vi "image.vi"() -> ()   [LabVIEW 2013]
uses:
  <vilib>/Analysis/Matrix/NI_Matrix.lvlib
  <vilib>/Utility/file.llb/Write To Spreadsheet File (DBL).vi
  <vilib>/Analysis/Matrix/Datatypes/RealMatrix.ctl
  <vilib>/Analysis/Matrix/Numeric/Conversions/Matrix To Array - RM.vi
  <vilib>/Utility/file.llb/Read From Spreadsheet File (DBL).vi
panel:
  in  "Normalize?":bool
  in  "Save The Cross Section":bool
  in  "ON":path=path "/Macintosh HD/Users/Ruchira/Desktop/scan1/ON1/Y-32_fit.txt"
  in  "OFF":path=path "/Macintosh HD/Users/Ruchira/Desktop/scan1/ON1/y_31_fit.txt"
  out "Intensity Graph":dbl[][](graph)=[[0.0999961901429774], [0.10000123166150422], [0.10000135033082976], [0.09999704994321655], [0.09999759071413349], [0.10000084663946385], [0.1000012117498761], [0.10000097689275309], [0.10000164876308568], [0.09999648287738241], [0.10000110689586153], [0.09999818237676397], [0.10000126793860856], [0.09999754550814881], [0.0999980392905063], [0.10000044482376341], [0.09999913803857505], [0.10000050220417034], [0.09999715423524554], [0.09999799513810394], [0.10000181351533373], [0.09999709728037659], [0.09999777905934876], [0.09999707127163737], [0.10000127901557891], [0.09999796410448629], [0.09999718267251918], [0.0999985636671887], [0.09999841240954438], [0.09999808500763945], [0.10000238691137875], [0.10000161846358738], [0.09999822930044115], [0.10000075848082599], [0.10000068933923355], [0.1000024236518158], [0.10000290568154932], [0.10000085686473831], [0.10000230225985311], [0.10000149836735855], [0.09999986636917042], [0.10000359405031024], [0.10000312564210484], [0.10000313147057305], [0.10000118234594123], [0.09999987554916473], [0.10000181684992422], [0.10000185606097113], [0.1000025842332808], [0.10000227930825865], [0.10000347944496162], [0.10000100625483241], [0.10000142101694179], [0.10000314994033971], [0.10000154469593482], [0.10000192220644337], [0.10000466479003443], [0.10000234032096383], [0.10000240345292899], [0.10000149911732752], [0.09999740374791438], [0.10000136412307498], [0.10000352573058052], [0.1000004648002058], [0.10000005079292161], [0.09999955770073203], [0.10000069450692534], [0.10000304014390352], [0.10000122773941927], [0.10000168512743678], [0.10000194792402127], [0.10000192695259297], [0.09999968237859753], [0.09999958623911322], [0.10000118777877205], [0.1000020603567743], [0.10000218588046038], [0.09999977985541698], [0.09999861297897399], [0.09999954403466309], [0.09999933084000477], [0.09999924980119886], [0.10000027299563718], [0.10000009189068723], [0.10000110682583423], [0.10000077949470162], [0.10000090534418594], [0.10000018726331182], [0.10000096980436052], [0.09999980494871381], [0.10000015878968854], [0.09999959204869212], [0.09999941000101689], [0.09999977355307214], [0.09999859679949125], [0.09999840143639106], [0.10000016454514019], [0.10000045652323415], [0.10000047732317208], [0.10000020087238798], [0.09999882340527957], [0.10000007126845203], [0.10000029214685592], [0.09999925931062281], [0.09999926329087266], [0.09999907646140645], [0.09999858993485494], [0.09999968917439243], [0.09999913973681834], [0.09999875844725434], [0.09999896445513062], [0.09999900543682053], [0.09999993071718452], [0.0999999102386502], [0.0999995214120633], [0.09999971735154342], [0.09999950486441825], [0.09999880162641392], [0.09999922584335166], [0.09999956823609847], [0.09999999668927682], [0.09999992113306001], [0.09999971240104609], [0.09999961415606441], [0.0999990191996489], [0.09999954251806992], [0.09999925150144613], [0.0999998365982448], [0.09999958671879616], [0.09999910599373554], [0.09999996361215446], [0.09999957627411026], [0.09999995030056676], [0.09999968902034741], [0.09999996957666005], [0.09999974435093766], [0.09999976482429569], [0.10000003037414487], [0.09999998475569946], [0.09999954938348765], [0.09999979074987307], [0.09999965366084819], [0.10000001991255952], [0.1000001850647135], [0.09999985563509438], [0.09999995855033227], [0.09999976121025504], [0.09999937741961164], [0.09999998666441115], [0.10000015954726275], [0.1000004123670828], [0.1000001063637803], [0.09999992798411764], [0.10000007921436647], [0.09999993517716374], [0.09999984988689666], [0.10000009355836353], [0.09999967891713826], [0.09999987103828216], [0.1000000712813875], [0.09999998747709593], [0.09999993295305948], [0.09999986632106737], [0.10000013745021331], [0.09999981188499174], [0.09999989255622112], [0.0999999919648023], [0.09999971354271445], [0.10000042793585165], [0.09999969311683246], [0.10000006809921125], [0.10000018404218568], [0.10000018015349744], [0.10000005384694884], [0.09999989767787482], [0.09999983532018687], [0.10000003722495465], [0.09999962269635267], [0.09999976172061785], [0.09999984532447814], [0.09999998784616544], [0.0999999039419567], [0.10000008441502968], [0.09999972051132222], [0.10000008779089652], [0.1000002890351282], [0.10000008731841208], [0.09999994222108334], [0.09999983237672086], [0.10000013421033312], [0.10000005141733095], [0.10000006535189712], [0.09999992565779832], [0.09999958959090645], [0.09999970593383432], [0.09999988681797735], [0.09999984714438878], [0.09999991710543132], [0.099999686490646], [0.0999998794498034], [0.09999985778736376]]
  in  "parameter Constrains":T1={"amp min"=-1.0, "amp max"=1.0, "center min"=600.0, "center max"=700.0, "FWHM min"=10.0, "FWHM max"=100.0, "offset min"=0.0, "offset max"=0.0}
  in  "File Format":u16(ring) items=["JPG", "PNG", "BMP"]
  in  "SigFig (micron)":dbl=1.0
  in  "Background Substract":bool=TRUE
  in  "Zoom Factor":sgl=1.0
  out "Picture":picture
  in  "path to bmp file":path=path "/Macintosh HD/Users/Ruchira/Desktop/ps.jpg"
  in  "Fitting Function":enum16{"Lorantzian", "fano", "gaussian"}(ring)=enum."gaussian"
  in  "Filter ?":bool=TRUE
  in  "?":u32(colorbox)=16715776
  in  "?":bool
  in  "?":u16(ring)=2 items=["", "Pick Spectrum ", "Fit Spectra", "Cross Section"]
  in  "?":bool
  in  "Fitting Directory":path=path "/Macintosh HD/Users/Ruchira/Desktop/scan1/ON1/Y_32_0/dia_1_X_39_4_Y_32_0_ON"
  in  "Initial \nparameters":dbl[](array[numeric])=[0.0, 0.1, 50.0, 183.0]
  out "Waveform Graph":cluster{"Array":dbl[]}[](graph)=[{"Array"=[0.999912, 1.0000062, 0.9999195, 1.0007249, 0.9996202, 0.9991244, 1.0002736, 0.9998005, 1.0002531, 1.0001882, 0.9997705, 0.9996142, 0.9994632, 0.9997326, 0.99964, 0.9993857, 1.0000215, 1.0006765, 0.9997504, 1.0006266, 0.9997772, 0.9992525, 1.0001104, 0.9999963, 0.9997144, 0.9990248, 0.99969, 0.9989677, 1.0008024, 0.9994781, 0.9996141, 0.9997979, 0.9997724, 0.9996542, 1.0000813, 0.9995505, 0.9997522, 0.9992789, 0.9997476, 1.0005772, 0.9997887, 0.9996226, 1.0004367, 1.0009052, 1.0000415, 0.9992441, 0.9992899, 0.9988662, 1.0001159, 0.9993691, 1.0000963, 0.998833, 0.9988622, 1.0002627, 0.9992917, 0.9994175, 0.9991441, 0.9992283, 0.9990043, 0.9988636, 1.0000361, 0.9996554, 0.9992461, 0.9990231, 0.999462, 0.9993146, 0.9997979, 1.0003636, 0.9998718, 0.999412, 0.9993142, 0.9986716, 0.9996698, 0.9993684, 0.9988869, 0.9991172, 1.0003158, 0.9997581, 1.0000962, 0.9996494, 0.9995781, 0.9989753, 0.9997771, 0.9995659, 0.9990109, 0.9994639, 0.9990328, 1.0002382, 0.9992761, 0.9996792, 0.9989703, 0.9994579, 0.9998822, 0.9984634, 0.9992488, 0.9996927, 0.9996856, 0.9999188, 0.9991421, 0.9996352, 0.9995514, 0.9994296, 0.9998158, 1.0003442, 0.9993032, 0.9998166, 0.9991794, 0.9992785, 0.9989296, 0.9992176, 0.9996715, 1.0002317, 0.9997447, 1.000023, 0.9999388, 1.0000318, 0.9993103, 0.9983221, 0.9997067, 0.9992942, 0.9994903, 1.000274, 0.9993993, 0.9996543, 0.9994589, 0.9987717, 0.9995216, 0.9996218, 0.9997857, 1.0003538, 1.0003287, 0.9998377, 1.0000575, 0.9994548, 0.999651, 1.000589, 0.9999774, 0.9998517, 0.9997108, 0.9997329, 0.9987114, 1.000017, 0.9998208, 0.9995178, 0.9995105, 0.9992935, 1.000017, 0.999771, 0.9997507, 0.9998368, 0.9989039, 0.9994854, 0.9991881, 0.9997416, 0.9995755, 0.9996139, 1.0004916, 0.9996789, 0.9997569, 1.0006737, 0.9995899, 0.9995284, 1.0003346, 0.9997696, 0.9997103, 0.9992941, 0.9995254, 0.9998266, 0.9995101, 0.999556, 0.9996889, 0.999612, 1.0004629, 0.9998417, 0.9998443, 0.9995054, 1.0001907, 0.999727, 1.0002715, 0.9998889, 0.9997173, 0.9996202, 0.9993741, 0.9997404, 0.9998444, 0.9995518, 0.9998645, 1.0002948, 0.9995542, 0.9993841, 0.9996716, 1.0003395, 0.9995428, 0.9992663, 0.9998679, 0.9990207, 0.9997029, 0.9999758, 1.0002127, 0.9991095, 0.9997171, 0.9994459, 0.9995794, 0.9996757, 0.9995238, 0.9992508, 0.9995349, 0.9996876, 0.9998513, 1.0002972, 1.0005107, 0.9995459, 0.9997344, 0.9993501, 0.998904, 0.9994265, 0.9996681, 0.9997693, 0.9998932, 1.0004375, 1.0003389, 0.9999753, 0.9999445, 1.0002389, 0.9992193, 1.0007039, 0.999621, 1.0005075, 0.9990674, 0.9989446, 0.9998963, 0.9995903, 0.999903, 0.9996576, 0.9997039, 0.9999802, 1.0004561, 0.9996246, 0.9994775, 1.0002422, 0.9993529, 1.0001368, 0.9998639, 1.0000355, 0.9992625, 0.9995799, 0.9999136, 0.9999445, 0.9994137, 1.0002099, 1.0002885, 0.9998356, 1.0008825, 1.0000316, 0.9999662, 0.9992243, 0.9998829, 1.0007041, 1.0002848, 0.9993363, 1.0001841, 1.0000274, 1.0003478, 1.0003174, 0.9999082, 1.0002834, 1.0002627, 0.9997852, 0.9991637, 1.0003098, 1.0002492, 1.0005535, 0.999675, 0.999759, 0.9995484, 1.0001614, 1.0000287, 1.0001989, 1.0004951, 1.0004172, 0.9999552, 0.9996557, 1.0003109, 0.9995099, 0.9997021, 0.9992045, 1.0007278, 0.9994112, 0.9999635, 0.9993279, 0.9996014, 1.0003337, 1.0000202, 0.9997986, 0.9991892, 0.9998672, 1.0000011, 0.9995615, 0.9991948, 0.9995186, 0.9998185, 0.9995575, 1.0000313, 0.9999638, 0.9999951, 1.0012059, 0.9997584, 1.0005391, 1.0011878, 1.000318, 0.9996395, 0.9996092, 0.9994599, 0.9997242, 1.0000628, 0.9993907, 0.9998052, 0.9995693, 1.0002239, 0.9993822, 0.9989864, 1.0008243000000001, 1.0008603, 1.000017, 0.99964, 0.9998918, 1.0009811, 0.9995773, 0.9999757, 0.9994455, 0.9999629, 0.9989937, 0.9993532, 0.9988021, 0.999775, 0.9994477, 1.0005354, 1.0004217, 0.9990068, 0.9990595, 0.999235, 0.9997253, 0.9999283, 1.0003691, 0.9987342, 0.9987156, 0.99932, 1.0006941, 0.9990174, 0.9995789, 1.0000781, 0.999864, 0.9987173, 0.9995567, 0.9998158, 0.9990578, 0.9997313, 0.9996173, 0.9997118, 1.0001294, 0.9995772, 0.9997848, 0.9992174, 1.0002083, 0.9998677, 0.999437, 0.9986994, 0.9989801, 0.9988885, 0.9988535, 0.9991101, 0.9993622, 1.0000297, 0.9998208, 0.9996366, 0.9999674, 0.9999051, 0.9994292, 0.9993126, 0.999776, 0.9990464, 0.9995287, 1.0005, 0.9994522, 0.9989594, 1.0000136, 0.998607, 0.9995734, 0.9998784, 0.9987946, 0.9995151, 0.9989061, 0.9996754, 0.9996827, 0.9990179, 0.9994808, 1.0005484, 0.9993381, 0.9996653, 0.9997457, 0.9998257, 0.9999206, 0.9996306, 0.9996981, 0.9994915, 1.000414, 0.9991374, 0.9999802, 0.9990244, 0.9995426, 0.9994226, 1.0005428, 0.9997184, 0.9996405, 0.9998817, 0.9990332, 0.999546, 0.9994692, 0.9995606, 0.999712, 1.0004374, 0.9985378, 1.0000077, 1.0013742, 0.9989422, 0.9999068, 0.999257, 0.9993879, 0.9996964, 1.0003505, 0.9998826, 0.9994893, 0.9999303, 1.000442, 1.0001266, 1.0005605, 0.9992218, 0.9994654, 0.9990975, 0.9999623, 0.9990798, 0.9998905, 0.9991768, 0.999592, 0.9999166, 0.9999282, 1.0001616, 1.0005988, 1.000266, 0.9993236, 1.0001337, 0.9993938, 0.9994889, 0.9982496, 1.0000666, 0.9995728, 0.9988732, 1.0000484, 0.9996128, 0.9998416, 0.9999103, 0.9994758, 0.9999986, 0.9992403, 0.9991495, 1.0000631, 0.9990761, 1.0002229, 1.0000052, 1.000004, 0.9996256, 1.0000775, 0.999592, 0.9997201, 0.9989163, 0.9989697, 1.0002479, 0.9999675, 0.999776, 0.9997987, 0.9994048, 0.9998939, 0.9997733, 0.9986924, 0.999714, 0.9994414, 1.0002745, 1.0000148, 0.9997425, 0.9995858, 1.0002273, 0.9996642, 1.0005309, 0.9997909, 0.9998647, 1.0004744, 0.9994365, 1.0003841, 1.0001789, 1.0003809, 0.9991066, 1.0002345, 1.0005149, 0.9986604, 1.0000528, 1.0003553, 0.9996183, 0.999854, 1.0004234, 0.9991074, 0.9999751, 0.9996607, 1.0001485, 1.00034, 0.9991534, 0.9996239, 0.9999622, 0.9999014, 0.9998442, 0.9994333, 0.9996824, 1.0012007, 0.9990924, 0.9996013, 0.9998479, 0.9997425, 0.9990558, 1.000082, 1.000111, 1.0005331, 1.0000641, 0.9994033, 1.0004079, 1.0001025, 1.0000838, 0.9990626, 1.0006284, 1.0000943, 1.000137, 0.9993611, 0.9996293, 1.0003729, 0.9998056, 1.0000649, 1.0002914, 0.9996269, 0.9997866, 0.9999594, 0.9997383, 0.9991266, 1.0001618, 0.9994388, 1.0002258, 0.9994914, 1.0000562, 0.9995762, 0.9998524, 0.9996511, 1.0010098, 0.9996345, 0.9992435, 0.9996726, 1.0001917, 1.0004534, 0.9996527, 0.9996541, 0.9994873, 0.998815, 0.9997382, 0.9989723, 0.9993279, 0.9988684, 1.0005942, 0.9979386, 0.9996604, 0.998509, 1.0000703, 0.999597, 0.9994641, 0.9995958, 0.999995, 0.9996274, 0.9998089, 0.9989087, 0.9996136, 1.0007132, 0.9995889, 0.99931, 0.9995004, 0.9986379, 0.99934, 0.9992054, 0.9991074, 1.0002335, 1.0002441, 0.999719, 0.9996165, 0.9997128, 0.998794, 0.9988396, 0.9998567, 0.9993354, 0.9993648, 0.9989801, 0.9996489, 0.9993824, 0.9998368, 0.9980654, 1.0000289, 0.9985257, 1.0002826, 0.999874, 0.9997462, 0.9995808, 0.9995395, 0.9988734, 0.9980803, 0.9995798, 1.00039, 0.9992561, 0.9996533, 0.9999288, 0.9985423, 0.9993574, 1.0003907, 0.9988179, 0.9996707, 0.9997962, 0.9988759, 1.0002284, 0.9996408, 0.9988728, 0.999683, 0.9994447, 1.0004125, 1.0008299, 0.9987556, 0.9992713, 0.9994446, 0.9983223, 0.9995367, 0.9980671, 0.9992592, 0.9998817, 0.9989496, 0.9996664, 1.000473, 0.9987348, 1.0003217, 0.9988259, 0.9988114, 1.0002154, 0.9995201, 0.9992665, 0.9992888, 0.9988897, 0.9986637, 0.9997617, 0.9991824, 0.998652, 0.999192, 0.9997019, 0.9985744, 0.9999023, 0.99976, 0.9989789, 0.9992547, 0.9985736, 1.0000799, 0.9994289, 1.000198, 1.0004209, 0.9995535, 0.9995055, 0.9999917, 0.9978965, 1.000103, 1.0002614, 0.9987275, 0.9997208, 0.9995843, 1.0004293, 0.9999196, 0.9997547, 0.9997684, 1.0000823, 0.9990606, 1.0000749, 1.0006261, 0.9992032, 1.0003915, 0.9986865, 0.9993972, 1.0006179, 0.999223, 0.9995273, 0.9999418, 0.9997804, 0.9990067, 0.9994214, 0.9988363, 0.9997792, 0.9992232, 0.9994337, 0.9996303, 0.9990614, 0.9987737, 0.9991485, 0.9999368, 0.9988097, 1.000023, 0.999718, 0.9993419, 0.9995108, 0.9988932, 0.9996122, 0.9996549, 0.9993274, 1.0007295, 0.9987502, 0.9991907, 1.000245, 0.9996555, 1.0001368, 0.9997992, 0.9998987, 0.9993079, 0.9997203, 1.0001504, 0.9991114, 0.9996201, 0.9997694, 0.998722, 0.9989102, 0.9998005, 0.9989434, 0.9990453, 1.0000478, 0.9993367, 0.9997115, 0.9999445, 0.998842, 0.9981667, 0.9997795, 0.9979156, 0.9987582, 0.9999457, 0.9985634, 0.9987168, 0.9989546, 0.9996025, 0.9987306, 0.9993737, 0.9990279, 0.9986008, 1.0004001, 0.9993854, 0.9993435, 0.9991244, 0.9991655, 0.9991997, 0.9996201, 0.999556, 0.9993827, 0.9996332, 0.9998294, 0.9992972, 0.9993395, 0.9992943, 0.9997331, 0.9996559, 0.9993133, 0.9997332, 1.0001546, 0.9998963, 0.9988493, 0.9982228, 0.9990334, 0.9996922, 0.999585, 0.99872, 0.9992144, 0.9997141, 0.998995, 1.0001988, 0.9992188, 0.9993191, 1.000408, 0.9996398, 0.9984199, 1.0003845, 0.9990073, 0.9987424, 0.9991647, 0.9990882, 1.0006108, 0.9996878, 0.9994017, 0.9997925, 0.9993464, 0.9995282, 1.0002015, 0.9995041, 0.9989298, 0.9996913, 0.998544, 0.9995248, 1.000274, 0.9993534, 0.9992568, 0.9998172, 0.9985249, 0.9998827, 0.9999777, 0.9996465, 0.9993267, 0.9985538, 0.9999634, 0.999692, 0.9998105, 0.9990786, 0.998777, 0.998742, 0.9994866, 0.9991291, 0.9991076, 0.9994755, 0.9993844, 0.9996325, 0.9997167, 0.9983325, 1.0000013, 1.0003206, 0.9993017, 1.0000534, 0.998928, 0.9992802, 1.0004163, 0.9985779, 0.9987091, 1.000012, 0.9995588, 0.9989666, 0.9986488, 0.9992081, 0.9996518, 1.0000042, 0.9990546, 0.9992699, 0.998815, 0.9993366, 0.9996229, 0.9992526, 0.9996555, 0.999927, 0.9989395, 1.0002995, 0.9994138, 0.9993524, 0.9989039, 0.9998021, 0.999467, 1.0003852, 0.9994779, 0.9991215, 1.0007633, 0.9992624, 0.999852, 0.999191, 0.9999406, 0.999067, 0.9998017, 0.9986019, 1.0000399, 0.9990516, 1.0003929, 0.9990066, 0.9995693, 0.9990149, 0.998768, 0.9999348, 0.9995828, 0.9993824, 0.9994241, 0.9989466, 0.9997066, 0.9991827, 1.0010118, 0.9997681, 0.9998445, 0.9988864, 0.9984717, 0.9995148, 0.9990124, 0.9994546, 0.9992063, 0.9994997, 0.9993552, 0.9985694, 0.9990449, 0.9988327, 0.9995954, 0.9989215, 0.9998563, 0.9991389, 0.9996583, 0.9996954, 0.9990346, 0.9989564, 0.9989618, 0.9990742, 0.9990664, 0.9993067, 0.999248, 0.9994816, 0.9991723, 0.9989503, 0.99956, 0.9992029, 0.9983765, 0.9996398, 0.9984304, 0.9994204, 1.0000248, 0.9995871, 0.9990603, 0.9995035, 0.9984536, 1.0001651, 1.0006427, 0.9989779, 0.9993951, 0.9994604, 0.9985639, 1.0000989, 0.998099, 0.9991217, 0.9990972, 0.999027, 0.9985814, 0.9985801, 0.9989235, 0.9996577, 0.9997086, 0.998898, 0.9996104, 0.9989361, 0.998648, 1.0002115, 0.9990118, 0.9988677, 0.9994482, 0.999177, 0.9990072, 0.9995065, 0.9993331, 0.9990698, 0.9986496, 0.9995377, 1.0006704, 0.9992097, 0.9987989, 0.9985685, 0.99976, 0.9987426, 0.9995563, 0.9991248, 0.9992443, 0.9989276, 0.9983766, 0.9994139, 0.9997891, 0.999956, 0.9992304, 0.9987388, 0.9984953, 0.999307, 0.9990246, 0.9988373, 0.9989017, 0.9991426, 0.9991718, 0.9992229, 0.9985943, 0.9989612, 0.9988095, 0.9995043, 0.9991213, 0.9993649, 0.9995521, 1.000257, 0.9991396, 0.9996828, 0.9988623, 0.9991661, 0.9982617, 0.9993377, 0.9976886, 1.0005162, 0.9987226, 0.9993491, 0.9984059, 0.998636, 0.999556, 0.9992717, 0.9984921, 0.999401, 0.9984477, 0.9991464, 1.0000037, 0.9990402, 0.9993154, 0.9992363, 0.9988391, 0.9996333, 0.9989477, 0.9992048, 1.0000735, 0.9992126, 0.9990736, 1.0003862, 0.9995333, 0.9994013, 0.9993385, 0.999072, 0.9992918, 0.9987017, 0.9996325, 0.9990081, 0.9996133, 0.9989096, 0.9989104, 0.9980355, 0.9995976, 0.9986304, 0.9988823, 0.9993512, 0.9986036, 0.9984648, 0.999202, 0.9995629, 0.9992173, 0.9987362, 0.9980147, 0.9998687, 0.9992276, 0.9989575, 0.998889, 0.9992327, 0.9991231, 0.9992699, 0.9997416, 0.9996087, 0.9996938, 0.9989509, 0.9993734, 0.9988294, 0.9991869, 0.9991652, 0.9986817, 0.999805, 0.9988091, 0.9987919, 0.9989816, 0.9995875, 0.9990158, 0.9986354, 0.9997111, 0.9997297, 0.9987274, 0.999885, 0.9991252, 0.9996094, 0.999989, 0.9991881, 0.9997831, 0.9996842, 0.9993126, 0.9997881, 0.9988679, 0.9990894, 0.9998617, 0.9991554, 0.9990344, 0.9992666, 0.9993193, 0.9999206, 0.9986974, 0.9992499, 1.0003586, 0.9988287, 0.9992303, 0.9998635, 0.9986143, 0.9980053, 1.0005758, 0.9976869, 0.9992939, 0.9987265, 0.9985804, 0.9985005, 0.9994571, 0.9989679, 0.9991719, 0.9984729, 0.9984019, 0.9995559, 0.9994761, 0.9997828, 0.9992282, 0.9989886, 0.9981934, 0.9990812, 0.998116, 0.9995994, 0.9989792, 0.9983792, 0.999598, 0.9988397, 0.9984028, 0.999649, 0.9988168, 0.9995654, 1.000411, 0.9986991, 0.9996752, 0.9986717, 0.9991131, 0.9988728, 0.9989572, 0.9981359, 0.9992972, 0.9988086, 0.9991376, 0.9990386, 0.9991565, 0.9990703, 0.9993521, 0.9986112, 1.0000715, 0.9986865, 0.9980398, 0.9988252, 0.9988827, 0.9982868, 0.999154, 0.9989643, 0.9991873, 0.998705, 0.9998231, 0.9993724, 0.9990766, 0.9987374, 0.9991775, 0.998257, 0.9984206, 1.0001665, 0.9987628, 0.9992235, 0.9991029, 0.9983892, 0.9999527, 0.9993111, 0.9989074, 0.999224, 0.9994221, 0.9993205, 0.9987931, 0.998174, 0.9995541, 0.9994415, 0.9990281, 0.9983542, 0.9989866, 0.999845, 0.9979003, 0.9987047, 0.9987763, 0.998873, 0.9986353, 0.9984925, 0.9996217, 0.9988643, 0.9993101, 0.9992636, 0.9995898, 0.9987621, 0.9981829, 0.9981291, 0.9994737, 0.9988985, 0.9992363, 1.0004459, 0.9985485, 0.9985508, 0.9995317, 0.9984561, 0.9987331, 0.9987794, 0.9995042, 0.999226, 0.9998977, 0.9990603, 0.9993281, 0.9987734, 0.9998663, 0.9993287, 0.9991301, 0.9994693, 0.9991984, 0.9985236, 0.9987384, 0.9990044, 0.9990008, 1.0001796, 1.0001622, 0.9985286, 0.9985244, 0.9981746, 0.9993868, 0.999581, 0.998385, 0.9992902, 0.9988528, 0.998681, 0.9995896, 0.998886, 0.9992045, 0.9996346, 0.9984278, 0.9989523, 1.00002, 0.9985499, 0.9997554, 0.9984731, 0.9991886, 0.9994447, 0.9995414, 0.9992294, 1.0000176, 0.9998677, 0.9994807, 0.9991572, 0.9990908, 0.9984204, 0.9988223, 0.9980823, 0.9985505, 0.9990276, 0.99854, 0.9989419, 0.9986103, 0.998692, 0.9997409, 0.9990202, 0.9985931, 0.9990757, 0.9986677, 0.9983732, 0.9987661, 0.9975218, 0.9997302, 0.9986096, 0.9995434, 0.9984961, 0.998689, 0.9990635, 1.0001033, 0.9988711, 0.9989773, 0.9990814, 0.9987169, 0.9997643, 0.9993714, 0.9989415, 0.9995076, 0.998517, 0.9990885, 0.9993318, 0.9976374, 0.9989427, 0.999286, 0.9980991, 0.9998433, 0.9994724, 0.9985809, 0.9993183, 0.999769, 0.9990847, 0.9984108, 0.9974821, 0.9993933, 0.9987865, 0.9981808, 0.9990092, 0.9997193, 0.9980069, 0.9985338, 0.9996889, 0.9992886, 0.9993596, 0.9988741, 0.9991357, 0.9992552, 0.9988415, 0.9988366, 0.9988451, 0.9985349, 0.9990692, 0.9997642, 0.9985883, 0.9992035, 0.9985753, 0.9986247, 0.9994766, 0.9993408, 0.9992854, 0.9986869, 0.9981718, 0.9987735, 0.9992385, 0.9986209, 0.9986522, 0.998752, 0.9987897, 0.9989516, 0.9991931, 0.9992246, 0.9994655, 0.9981522, 0.9995083, 0.9988177, 0.9984444, 0.9998394, 0.998757, 0.998562, 0.9994411, 0.9988745, 0.9988899, 0.9991615]}]
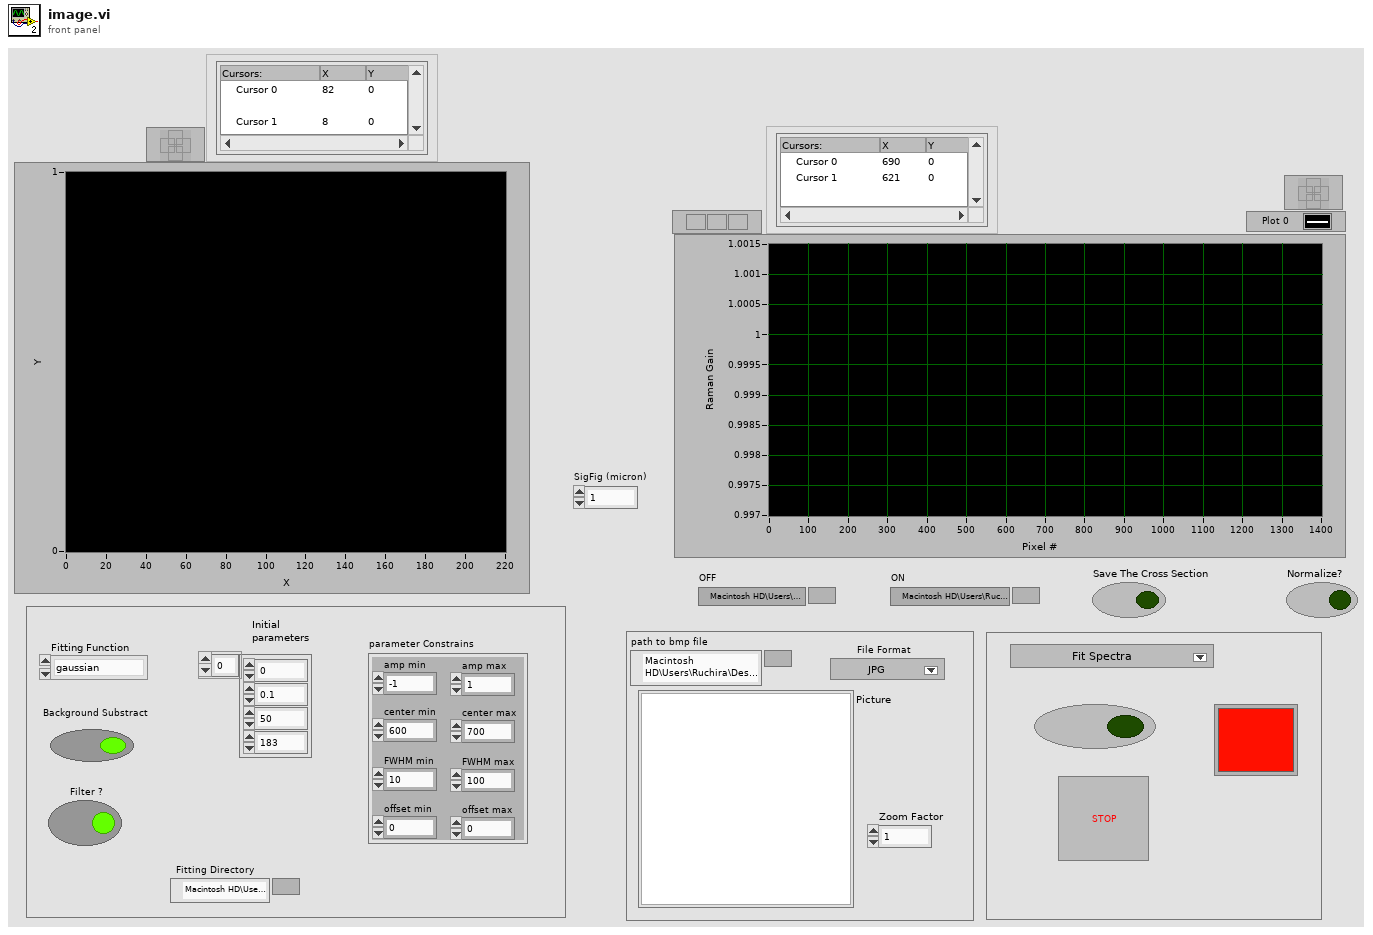
[diagram p1: front panel]
types:
  T1 = cluster{"amp min":dbl, "amp max":dbl, "center min":dbl, "center max":dbl, "FWHM min":dbl, "FWHM max":dbl, "offset min":dbl, "offset max":dbl}
  T2 = cluster{string[], "all rows":dbl[][], i32[], i32[], "size":i64}
  T3 = typedef "NI_Matrix.lvlib/RealMatrix.ctl" = dbl[][]
  T4 = typedef "imagedata.ctl" = cluster{"image type":i32, "image depth":i32, "image":u8[], "mask":u8[], "colors":u32[], "Rectangle":cluster{"left":i16, "top":i16, "right":i16, "bottom":i16}}
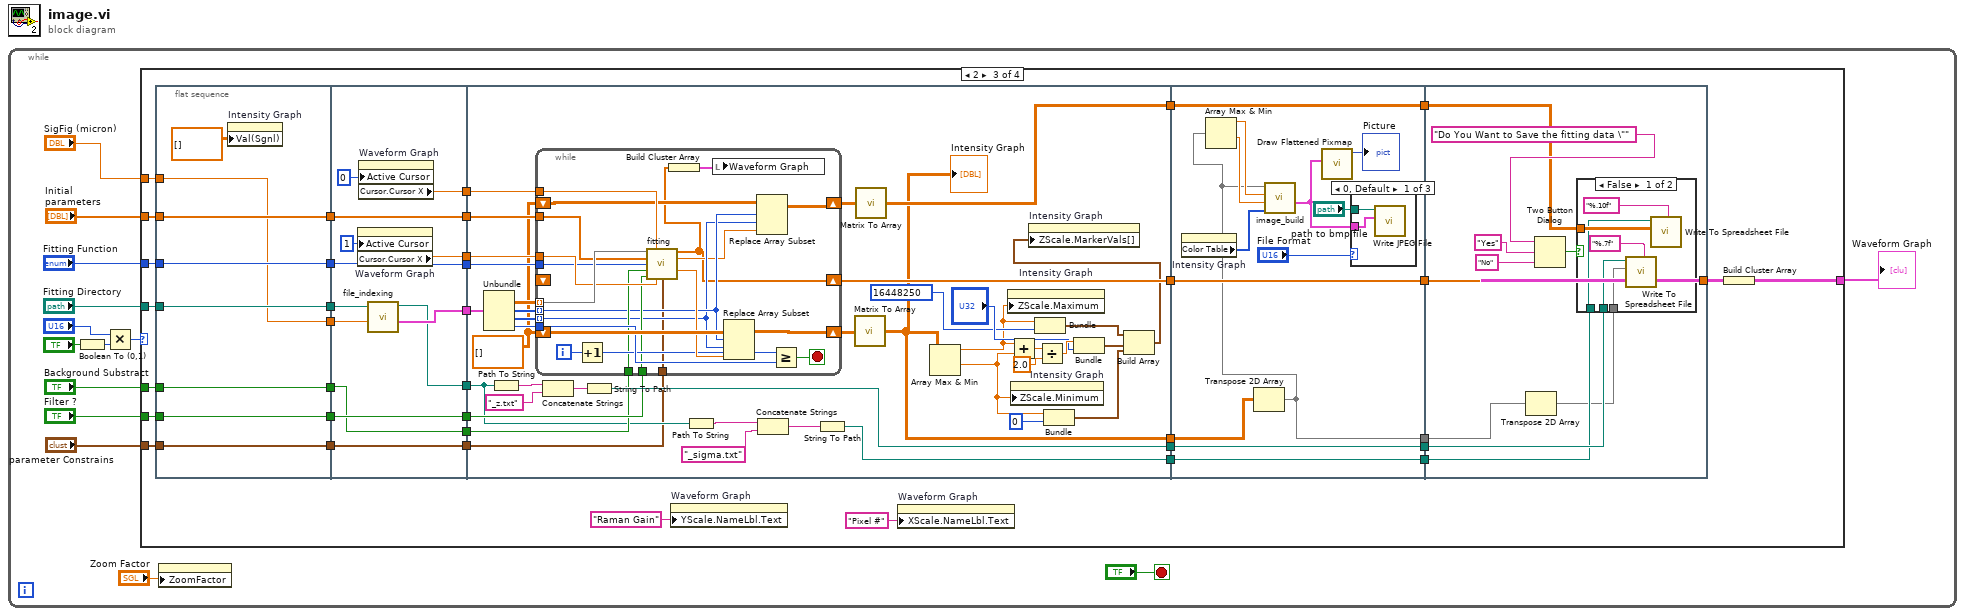
[diagram p0: block diagram]
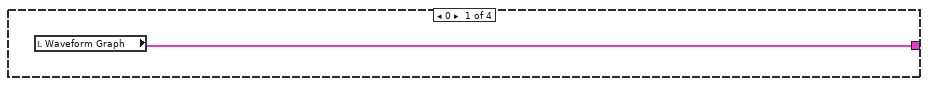
[diagram p2: hidden frame]
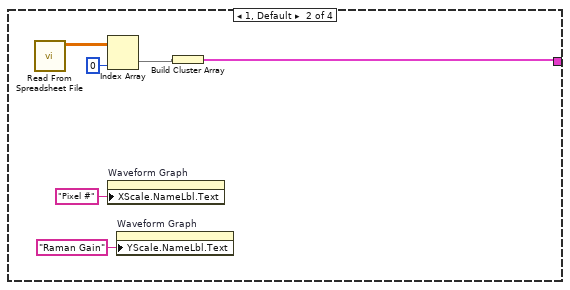
[diagram p3: hidden frame]
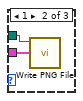
[diagram p4: hidden frame]
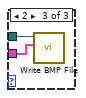
[diagram p5: hidden frame]
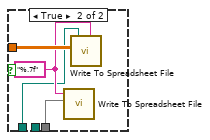
[diagram p6: hidden frame]
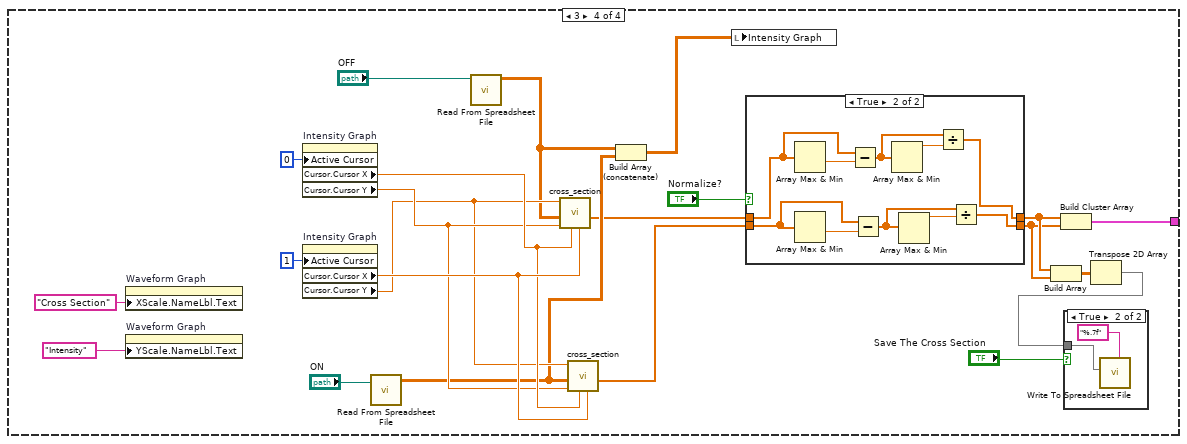
[diagram p7: hidden frame]
diagram:
  n1 = while {
    stop <- "?" stop-if-true
    n2 = Boolean To (0,1)(Boolean="?") -> (0, 1=w11:i16)
    n3 = Multiply(x="?", y=w11) -> (x*y=w10:u16)
    n4 = case shown="2" w10 {
      tunnel: [w15 w16 w22 w183] -> w14
      tunnel: "Fitting Directory" -> [_ _ w57 _]
      tunnel: "Filter ?" -> [_ _ w50 _]
      tunnel: "Fitting Function" -> [_ _ w47 _]
      tunnel: "Initial \nparameters" -> [_ _ w44 _]
      tunnel: "Background Substract" -> [_ _ w36 _]
      tunnel: "SigFig (micron)" -> [_ _ w33 _]
      tunnel: "parameter Constrains" -> [_ _ w26 _]
      frame 0 {
        n5 = local read "Waveform Graph"() -> (w15:cluster{"Array":dbl[]}[])
      }
      frame 1, Default {
        n6 = call-poly <vilib>:"Read From Spreadsheet File.vi"() -> ("all rows"=w21:dbl[][])  [unwired: 7 in, 4 out]
        n7 = Index Array(array=w21, index (col)=0 ("disabled index (col)")) -> (element=w17:dbl[])  [unwired: 1 in]
        n8 = property on="Waveform Graph" class="WFGraph (strict)"("XScale.NameLbl.Text"="Pixel #" ("X Scale.Name Label.Text")) -> ()  [unwired: 2 in, 2 out]
        n9 = property on="Waveform Graph" class="WFGraph (strict)"("YScale.NameLbl.Text"="Raman Gain" ("Y Scale.Name Label.Text")) -> ()  [unwired: 2 in, 2 out]
        n10 = Build Cluster Array(w17) -> (w16:cluster{"all rows":dbl[]}[])
      }
      frame 2 {
        n11 = flat-sequence {
          tunnel: w57 -> [w66]
          tunnel: [w66] -> w53
          tunnel: [w64] -> w51
          tunnel: w50 -> [w64]
          tunnel: [w62] -> w48
          tunnel: w47 -> [w62]
          tunnel: [w63] -> w45
          tunnel: w44 -> [w63]
          tunnel: [w61] -> w37
          tunnel: w36 -> [w61]
          tunnel: [w60] -> w34
          tunnel: w33 -> [w60]
          tunnel: [w59] -> w27
          tunnel: w26 -> [w59]
          tunnel: [w74] -> w58
          tunnel: [w78] -> w56
          tunnel: [w77] -> w55
          tunnel: [w73] -> w54
          tunnel: w53 -> [w75]
          tunnel: [w72] -> w52
          tunnel: w51 -> [w72]
          tunnel: [w71] -> w49
          tunnel: w48 -> [w71]
          tunnel: [w70] -> w46
          tunnel: w45 -> [w70]
          tunnel: w37 -> [w69]
          tunnel: [w69] -> w35
          tunnel: w34 -> [w68]
          tunnel: [w67] -> w28
          tunnel: w27 -> [w67]
          tunnel: w58 -> [w118]
          tunnel: w56 -> [w112]
          tunnel: w55 -> [w111]
          tunnel: w54 -> [w87]
          tunnel: [w107] -> w43
          tunnel: [w80] -> w41
          tunnel: [w99] -> w39
          tunnel: w52 -> [w95]
          tunnel: w49 -> [w94]
          tunnel: w46 -> [w93]
          tunnel: w35 -> [w92]
          tunnel: [w81] -> w31
          tunnel: [w86] -> w30
          tunnel: w28 -> [w84]
          tunnel: w43 -> [w153]
          tunnel: [w153] -> w42
          tunnel: w41 -> [w142]
          tunnel: [w141] -> w40
          tunnel: w39 -> [w152]
          tunnel: [w152] -> w38
          tunnel: [w144] -> w32
          tunnel: w31 -> [w144]
          tunnel: w30 -> [w143]
          tunnel: [w143] -> w29
          tunnel: [w169] -> w23
          tunnel: w42 -> [w169]
          tunnel: w40 -> [w161]
          tunnel: w38 -> [w163]
          tunnel: w32 -> [w164]
          tunnel: w29 -> [w162]
          frame #0 {
            n12 = property on="Intensity Graph" class="IntGraph (strict)"("Val(Sgnl)"=dbl[][] [] ("Value (Signaling)")) -> ()  [unwired: 2 in, 2 out]
          }
          frame #1 {
            n13 = property on="Waveform Graph" class="WFGraph (strict)"("Active Cursor"=u32 1) -> ("Cursor.Cursor X"=w78:dbl)  [unwired: 2 in, 2 out]
            n14 = property on="Waveform Graph" class="WFGraph (strict)"("Active Cursor"=u32 0) -> ("Cursor.Cursor X"=w77:dbl)  [unwired: 2 in, 2 out]
            n15 = call "file_indexing.vi"("Sigfig"=w68, "path"=w75) -> ("output cluster"=w74:T2, "stripped path"=w73:path)  [unwired: 7 in]
          }
          frame #2 {
            w90 = T3 [] ("Real Matrix")
            n16 = Unbundle(w118) -> ("all rows"=w117:dbl[][], w115:i32[], w116:i32[], "size"=w114:i64)  [unwired: 1 out]
            n17 = Path To String(path=w87) -> (string=w110:string)
            n18 = while {
              tunnel: w117 -> [w140] mode=indexing
              shift-right: [w119] -> w107
              shift-left: _ -> [_]
              shift-right: [w138] -> w113
              shift-left: w90 -> [w137]
              tunnel: w116 -> [w125] mode=indexing
              tunnel: w115 -> [w126] mode=indexing
              tunnel: w114 -> [w136]
              tunnel: w112 -> [w132]
              tunnel: w111 -> [w131]
              tunnel: w95 -> [w130]
              tunnel: w94 -> [w129]
              tunnel: w93 -> [w128]
              tunnel: w92 -> [w127]
              shift-right: [w124] -> w89
              shift-left: w90 -> [w123]
              tunnel: w84 -> [w121]
              i -> [w134]
              stop <- w139 stop-if-true
              n19 = Increment(x=w134) -> (x+1=w133:i32)
              n20 = call "fitting.vi"("array"=w140, "x"=w131, "initial parameters"=w128, "Enum"=w129, "Background"=w127, "Filter"=w130, "x 2"=w132, "parameter bounds"=w121) -> ("array 2"=w119:dbl[], "standard deviation"=w122:dbl, "Fitting"=w135:dbl)  [unwired: 3 in, 2 out]
              n21 = Build Cluster Array(w119) -> (w120:cluster{"array 2":dbl[]}[])
              n22 = local write "Waveform Graph"(w120) -> ()
              n23 = Replace Array Subset(array=w137, new element=w135, index (row)=w126, index (col)=w125) -> (w138:T3)
              n24 = Replace Array Subset(array=w123, new element=w122, index (row)=w126, index (col)=w125) -> (w124:T3)
              n25 = Greater Or Equal?(x=w133, y=w136) -> (x >= y?=w139:bool)
            }
            n26 = Concatenate Strings(w110, "_z.txt" ("string")) -> (w108:string)
            n27 = String To Path(string=w108) -> (path=w99:path)
            n28 = Path To String(path=w87) -> (string=w83:string)
            n29 = Concatenate Strings(w83, "_sigma.txt" ("string")) -> (w88:string)
            n30 = String To Path(string=w88) -> (path=w86:path)
            n31 = call-poly <vilib>:"Matrix To Array.vi"("Real Matrix"=w113) -> ("Real 2D Array"=w80:dbl[][])
            "Intensity Graph" <- w80
            n32 = call-poly <vilib>:"Matrix To Array.vi"("Real Matrix"=w89) -> ("Real 2D Array"=w81:dbl[][])
            n33 = Array Max & Min(array=w80) -> (max value=w91:dbl, min value=w85:dbl)  [unwired: 2 out]
            n34 = property on="Intensity Graph" class="IntGraph (strict)"("ZScale.Maximum"=w91) -> ()  [unwired: 2 in, 2 out]
            n35 = Add(x=w91, y=w85) -> (x+y=w103:dbl)
            n36 = property on="Intensity Graph" class="IntGraph (strict)"("ZScale.Minimum"=w85) -> ()  [unwired: 2 in, 2 out]
            n37 = Bundle(w91, 16448250) -> (w105:cluster{dbl, i32})  [unwired: 1 in]
            n38 = Divide(x=w103, y=2.0) -> (x/y=w100:dbl)
            n39 = Bundle(w85, 0) -> (w104:cluster{dbl, i32})  [unwired: 1 in]
            n40 = Bundle(w100, "?") -> (w101:cluster{dbl, u32})  [unwired: 1 in]
            n41 = Build Array(w105, w101, w104) -> (w98:cluster{dbl, u32}[])
            n42 = property on="Intensity Graph" class="IntGraph (strict)"("ZScale.MarkerVals[]"=w98) -> ()  [unwired: 2 in, 2 out]
          }
          frame #3 {
            n43 = property on="Intensity Graph" class="IntGraph (strict)"() -> ("Color Table"=w151:u32[])  [unwired: 2 in, 2 out]
            n44 = Transpose 2D Array(2D array=w142) -> (transposed array=w141:dbl[][])
            n45 = Array Max & Min(array=w141) -> (max value=w149:dbl, min value=w148:dbl)  [unwired: 2 out]
            n46 = call "image_build.vi"("colors"=w151, "Min"=w148, "Max"=w149, "Data"=w141) -> ("image data"=w145:T4)  [unwired: 7 in]
            n47 = call <vilib>:"Draw Flattened Pixmap.vi"("image data"=w145) -> ("new picture"=→"Picture":picture)  [unwired: 8 in]
            n48 = case shown="0, Default" "File Format" {
              tunnel: "path to bmp file" -> [w155 w156 w158]
              tunnel: w145 -> [w154 w157 w159]
              frame 0, Default {
                n49 = call <vilib>:"Write JPEG File.vi"("image data"=w154, "path to JPEG file"=w155) -> ()  [unwired: 8 in, 2 out]
              }
              frame 1 {
                n50 = call <vilib>:"Write PNG File.vi"("image data"=w157, "path to PNG file"=w156) -> ()  [unwired: 8 in, 2 out]
              }
              frame 2 {
                n51 = call <vilib>:"Write BMP File.vi"("image data"=w159, "path to BMP file"=w158) -> ()  [unwired: 8 in, 2 out]
              }
            }
          }
          frame #4 {
            n52 = Transpose 2D Array(2D array=w161) -> (transposed array=w160:dbl[][])
            n53 = Two Button Dialog(message="Do You Want to Save the fitting data \"", 1:"No" ("F button name (\"Cancel\")"), 2:"Yes" ("T button name (\"OK\")")) -> (T button?=w165:bool)
            n54 = case shown="False" w165 {
              tunnel: w160 -> [w174 w179]
              tunnel: w163 -> [w175 _]
              tunnel: w164 -> [w173 w178]
              tunnel: w162 -> [w172 w176]
              frame False {
                n55 = call-poly <vilib>:"Write To Spreadsheet File.vi"("format (%.3f)"="%.7f", "2D data"=w174, "file path (dialog if empty)"=w175) -> ()  [unwired: 5 in, 1 out]
                n56 = call-poly <vilib>:"Write To Spreadsheet File.vi"("format (%.3f)"="%.10f", "2D data"=w173, "file path (dialog if empty)"=w172) -> ()  [unwired: 5 in, 1 out]
              }
              frame True {
                w177 = "%.7f" ("format (%.3f)")
                n57 = call-poly <vilib>:"Write To Spreadsheet File.vi"("format (%.3f)"=w177, "2D data"=w179) -> ()  [unwired: 6 in, 1 out]
                n58 = call-poly <vilib>:"Write To Spreadsheet File.vi"("format (%.3f)"=w177, "2D data"=w178, "file path (dialog if empty)"=w176) -> ()  [unwired: 5 in, 1 out]
              }
            }
          }
        }
        n59 = property on="Waveform Graph" class="WFGraph (strict)"("YScale.NameLbl.Text"="Raman Gain" ("Y Scale.Name Label.Text")) -> ()  [unwired: 2 in, 2 out]
        n60 = property on="Waveform Graph" class="WFGraph (strict)"("XScale.NameLbl.Text"="Pixel #" ("X Scale.Name Label.Text")) -> ()  [unwired: 2 in, 2 out]
        n61 = Build Cluster Array(w23) -> (w22:cluster{"array 2":dbl[]}[])
      }
      frame 3 {
        n62 = property on="Waveform Graph" class="WFGraph (strict)"("XScale.NameLbl.Text"="Cross Section" ("X Scale.Name Label.Text")) -> ()  [unwired: 2 in, 2 out]
        n63 = property on="Waveform Graph" class="WFGraph (strict)"("YScale.NameLbl.Text"="Intensity" ("Y Scale.Name Label.Text")) -> ()  [unwired: 2 in, 2 out]
        n64 = property on="Intensity Graph" class="IntGraph (strict)"("Active Cursor"=u32 0) -> ("Cursor.Cursor X"=w195:dbl, "Cursor.Cursor Y"=w194:dbl)  [unwired: 2 in, 2 out]
        n65 = property on="Intensity Graph" class="IntGraph (strict)"("Active Cursor"=u32 1) -> ("Cursor.Cursor X"=w196:dbl, "Cursor.Cursor Y"=w193:dbl)  [unwired: 2 in, 2 out]
        n66 = call-poly <vilib>:"Read From Spreadsheet File.vi"("file path (dialog if empty)"="ON") -> ("all rows"=w190:dbl[][])  [unwired: 6 in, 4 out]
        n67 = call-poly <vilib>:"Read From Spreadsheet File.vi"("file path (dialog if empty)"="OFF") -> ("all rows"=w191:dbl[][])  [unwired: 6 in, 4 out]
        n68 = call "cross_section.vi"("X2"=w196, "X1"=w195, "Y1"=w194, "array"=w191, "Y2"=w193) -> ("Array"=w186:dbl[])  [unwired: 6 in]
        n69 = call "cross_section.vi"("X2"=w196, "X1"=w195, "Y1"=w194, "array"=w190, "Y2"=w193) -> ("Array"=w185:dbl[])  [unwired: 6 in]
        n70 = Build Array (concatenate)(w191, w190) -> (w184:dbl[][])
        n71 = local write "Intensity Graph"(w184) -> ()
        n72 = case shown="True" "Normalize?" {
          tunnel: w186 -> [w202 w210]
          tunnel: w185 -> [w203 w211]
          tunnel: [w202 w205] -> w182
          tunnel: [w203 w204] -> w181
          frame False {
          }
          frame True {
            n73 = Array Max & Min(array=w210) -> (min value=w213:dbl)  [unwired: 3 out]
            n74 = Array Max & Min(array=w211) -> (min value=w212:dbl)  [unwired: 3 out]
            n75 = Subtract(x=w210, y=w213) -> (x-y=w208:dbl[])
            n76 = Subtract(x=w211, y=w212) -> (x-y=w206:dbl[])
            n77 = Array Max & Min(array=w208) -> (max value=w209:dbl)  [unwired: 3 out]
            n78 = Array Max & Min(array=w206) -> (max value=w207:dbl)  [unwired: 3 out]
            n79 = Divide(x=w208, y=w209) -> (x/y=w205:dbl[])
            n80 = Divide(x=w206, y=w207) -> (x/y=w204:dbl[])
          }
        }
        n81 = Build Array(w182, w181) -> (w189:dbl[][])
        n82 = Build Cluster Array(w182, w181) -> (w183:cluster{"Array":dbl[]}[])
        n83 = Transpose 2D Array(2D array=w189) -> (transposed array=w180:dbl[][])
        n84 = case shown="True" "Save The Cross Section" {
          tunnel: w180 -> [_ w214]
          frame False {
          }
          frame True {
            n85 = call-poly <vilib>:"Write To Spreadsheet File.vi"("format (%.3f)"="%.7f", "2D data"=w214) -> ()  [unwired: 6 in, 1 out]
          }
        }
      }
    }
    "Waveform Graph" <- w14
    n86 = property on="Picture" class="Pict"("ZoomFactor"="Zoom Factor") -> ()  [unwired: 2 in, 2 out]
  }
